vi "set_value.vi"(8 "error in (no error)":errorcluster, 10 "mlir.lvlib:SsaId.lvclass":refnum<class "SsaId.lvclass">, 11 "OpResult in":refnum<class "OpResult.lvclass">) -> (0 "error out":errorcluster, 3 "OpResult out":refnum<class "OpResult.lvclass">)   [LabVIEW 2020, in "mlir.lvlib" / "OpResult.lvclass"]
uses:
  OpResult.lvclass
  SsaId/SsaId.lvclass
  OpResult.lvclass/OpResult.ctl
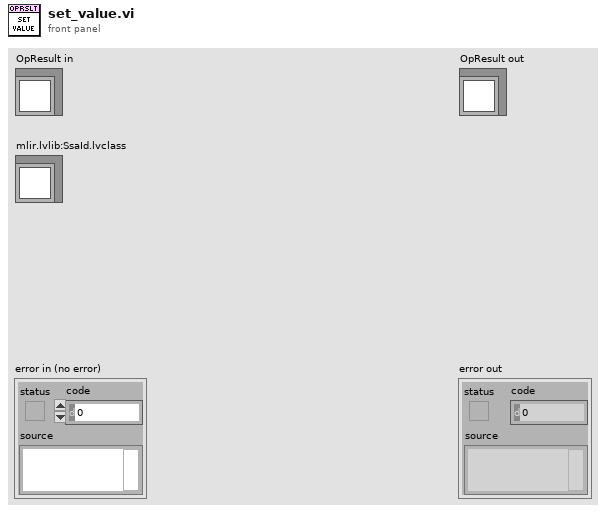
[diagram p1: front panel]
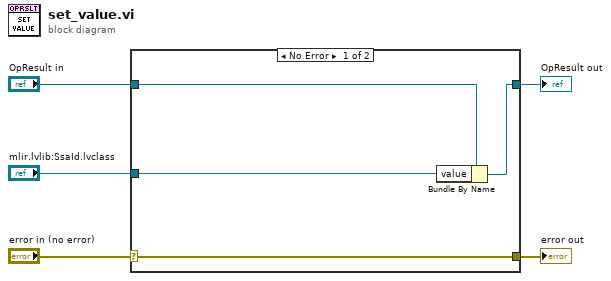
[diagram p0: block diagram]
diagram:
  n1 = case shown="No Error" "error in (no error)" {
    selector: "error in (no error)" -> [w9 w10]
    tunnel: [w9 w10] -> w4
    tunnel: [w7 w11] -> w2
    tunnel: "OpResult in" -> [w8 w11]
    tunnel: "mlir.lvlib:SsaId.lvclass" -> [w6 _]
    frame No Error {
      n2 = Bundle By Name(cluster=w8, "value"=w6) -> (w7:refnum<class "OpResult.lvclass">)
    }
    frame Error {
    }
  }
  "error out" <- w4
  "OpResult out" <- w2
